vi "Convex Hull.vi"(3 "Sorted Array":T1[](array[typedef])) -> (0 "Interior Points":T1[](array[typedef]), 1 "Convex Hull":T1[](array[typedef]))   [LabVIEW 2018]
uses:
  Graham Scan Point.ctl
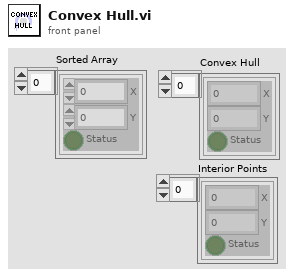
[diagram p1: front panel]
types:
  T1 = typedef "Graham Scan Point.ctl" = cluster{"X":i32, "Y":i32, "Status":bool}
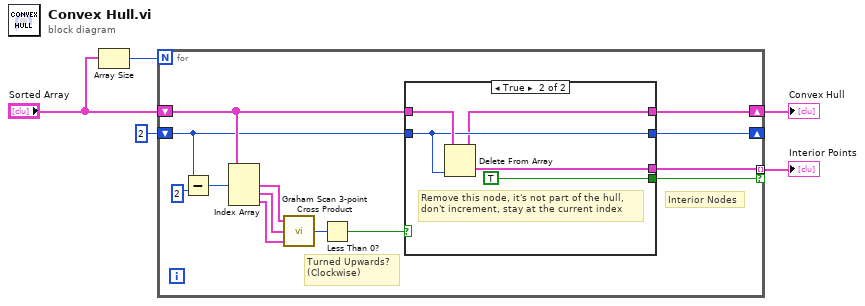
[diagram p0: block diagram]
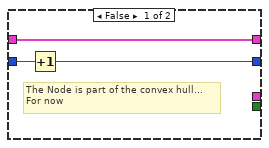
[diagram p2: hidden frame]
diagram:
  n1 = Array Size(array="Sorted Array") -> (size(s)=w4:i32)
  n2 = for {
    N: w4 -> [_]
    shift-right: [w10] -> w5
    shift-left: "Sorted Array" -> [w11]
    shift-right: [w8] -> _
    shift-left: 2 -> [w9]
    tunnel: [w7] -> w1 mode=indexing if=w6
    # "Interior Nodes"
    # "Turned Upwards?\n(Clockwise)"
    n3 = Subtract(x=w9, y=2) -> (x-y=w17:i32)
    n4 = Index Array(array=w11, index #1=w17) -> (element #1=w16:T1, element #2=w15:T1, element #3=w14:T1)  [unwired: 2 in]
    n5 = call "Graham Scan 3-point Cross Product.vi"("C"=w14, "B"=w15, "A"=w16) -> ("|| AB X AC ||"=w13:i32)
    n6 = Less Than 0?(x=w13) -> (x < 0?=w12:bool)
    n7 = case shown="True" w12 {
      tunnel: w11 -> [w21 w26]
      tunnel: [w21 w24] -> w10
      tunnel: w9 -> [w20 w25]
      tunnel: [w19 w25] -> w8
      tunnel: [_ w23] -> w7
      tunnel: [_ TRUE] -> w6
      frame False {
        # "The Node is part of the convex hull...\nFor now"
        n8 = Increment(x=w20) -> (x+1=w19:i32)
      }
      frame True {
        # "Remove this node, it's not part of the hull,\ndon't increment, stay at the current index"
        n9 = Delete From Array(array=w26, index=w25) -> (deleted portion=w23:T1, array with subset deleted=w24:T1[])  [unwired: 1 in]
      }
    }
  }
  "Convex Hull" <- w5
  "Interior Points" <- w1
